vi "GE5565 Status.vi"(4 "error in (no error)":errorcluster, 7 "VMIC reference in":T1) -> (0 "error out":errorcluster, 2 "Node ID":u8, 3 "VMIC reference out":T1)   [LabVIEW 2019, in "GE_RM_Real Time.lvlib"]
uses:
  GE_RM_Real Time.lvlib
  <vilib>/Instr/_visa.llb/VISA Register Access Address Space.ctl
panel:
  out "Data bin":u32 format="%032b"
  out "Data":u32
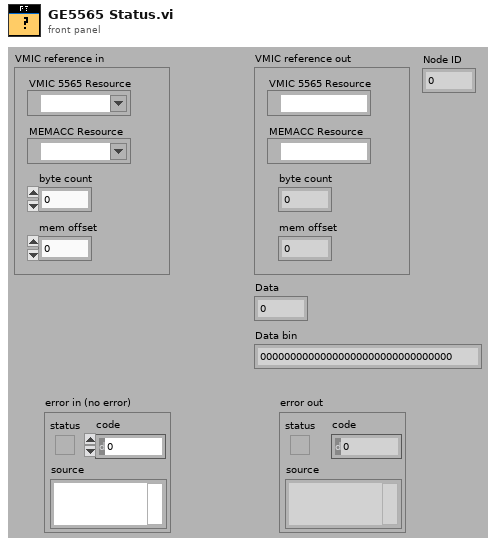
[diagram p1: front panel]
types:
  T1 = cluster{"VMIC 5565 Resource":refnum<visa-resource-name>, "MEMACC Resource":refnum<visa-resource-name>, "byte count":u32, "mem offset":u32}
  T2 = typedef "VISA Register Access Address Space.ctl" = u16
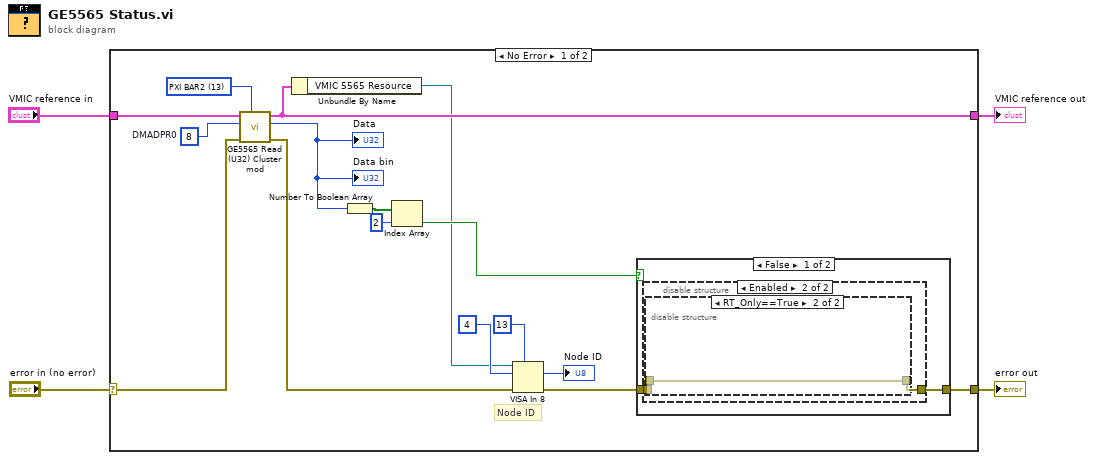
[diagram p0: block diagram]
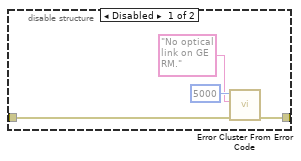
[diagram p2: hidden frame]
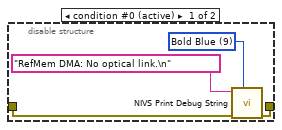
[diagram p3: hidden frame]
diagram:
  n1 = case shown="No Error" "error in (no error)" {
    selector: "error in (no error)" -> [w19 w35]
    tunnel: "VMIC reference in" -> [w20 w36]
    tunnel: [w9 w36] -> w1
    tunnel: [w15 w35] -> w3
    frame No Error {
      w17 = u32 8  # DMADPR0
      w18 = T2 13 items=["VXI/VME A16"=1, "VXI/VME A24"=2, "VXI/VME A32"=3, "VXI/VME A64"=4, "PXI Memory Allocations"=9, "PXI Configuration"=10, "PXI BAR0"=11, "PXI BAR1"=12, "PXI BAR2"=13, "PXI BAR3"=14, "PXI BAR4"=15, "PXI BAR5"=16] ("Address Space")
      # "Node ID"
      n2 = call "GE5565 Read (U32) Cluster mod.vi"("Address Space"=w18, "error in (no error)"=w19, "offset (0)"=w17, "VMIC reference in"=w20) -> ("error out"=w6:errorcluster, "Data"=w16:u32, "VMIC reference out"=w9:T1)  [unwired: 5 in]
      "Data" <- w16
      "Data bin" <- w16
      n3 = Unbundle By Name(w9) -> ("VMIC 5565 Resource"=w8:refnum<visa-resource-name>)
      n4 = Number To Boolean Array(number=w16) -> (Boolean array=w14:bool[])
      n5 = Index Array(array=w14, index=2) -> (element=w12:bool)
      n6 = VISA In 8(7:u16 13 ("BAR2"), 8:w6, 10:u32 4 ("Node ID Register"), 11:w8) -> (0:w7:errorcluster, 2:→"Node ID":u8)  [unwired: 1 out]
      n7 = case shown="False" w12 {
        tunnel: w7 -> [w22 w34]
        tunnel: [w21 w34] -> w15
        frame False {
          n8 = disable-structure shown="Enabled" {
            disable-tunnel: w22 -> [w26 w28]
            disable-tunnel: [w25 w27] -> w21
            frame Disabled {
              n9 = call <vilib>:"Error Cluster From Error Code.vi"("error in (no error)"=w26, "error message (\"\")"="No optical  link on GE RM." ("error message (\"\")"), "error code (0)"=5000) -> ("error out"=w25:errorcluster)  [unwired: 6 in]
            }
            frame Enabled {
              n10 = disable-structure shown="RT_Only==True" {
                disable-tunnel: w28 -> [w31 w33]
                disable-tunnel: [w30 w33] -> w27
                frame condition #0 (active) {
                  w32 = u16 9 items=["Plain White"=7, "Bold White"=15, "Bold Blue"=9, "Bold Green"=10, "Bold Red"=12] ("Color (Plain White)")
                  n11 = call "NIVS Print Debug String.vi"("Color (Plain White)"=w32, "error in (no error)"=w31, "Debug String"="RefMem DMA: No optical link.\n") -> ("error out"=w30:errorcluster)  [unwired: 7 in]
                }
                frame condition #1 {
                }
              }
            }
          }
        }
        frame True {
        }
      }
    }
    frame Error {
    }
  }
  "error out" <- w3
  "VMIC reference out" <- w1
